vi "SaveImage.vi"(8 "error in (no error)":errorcluster caption="错误输入（无错误）", 9 "pSaveParam In":T1, 10 "pDstBuffer In":u8[](array[numeric]), 11 "pSrcData":u8[](array[numeric])) -> (0 "error out":errorcluster caption="错误输出", 1 "pSaveParam Out":T1, 2 "pDstBuffer Out":u8[](array[numeric]), 3 "function return":i32)   [LabVIEW 2015, in "MvCameraControl.lvlib"]
doc: "MV_LV_API int __stdcall SaveImage(MV_SAVE_IMAGE_PARAM* pSaveParam);"
uses:
  MvCameraControl.lvlib
  MvCameraPatch.dll
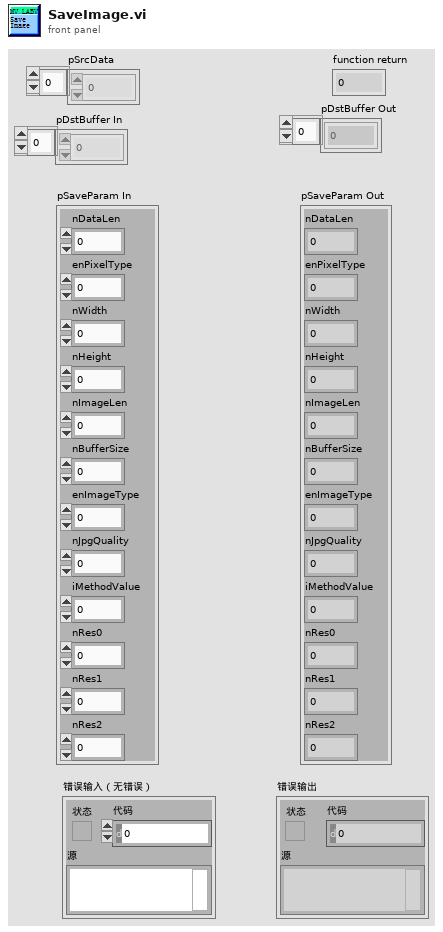
[diagram p1: front panel]
types:
  T1 = cluster{"nDataLen":u32, "enPixelType":i32, "nWidth":u16, "nHeight":u16, "nImageLen":u32, "nBufferSize":u32, "enImageType":u32, "nJpgQuality":u32, "iMethodValue":u32, "nRes0":u32, "nRes1":u32, "nRes2":u32}
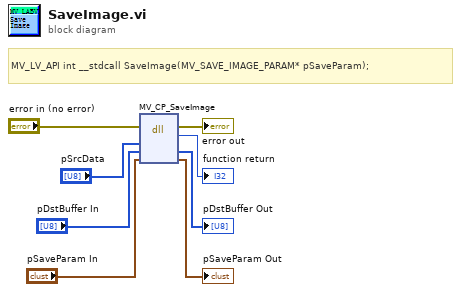
[diagram p0: block diagram]
diagram:
  # "MV_LV_API int __stdcall SaveImage(MV_SAVE_IMAGE_PARAM* pSaveParam);"
  n1 = dll-call lib="MvCameraPatch.dll" fn="MV_CP_SaveImage"(error in="error in (no error)", "pSrcData"="pSrcData", "pDstBuffer"="pDstBuffer In", "pSaveParam Out"="pSaveParam In") -> (error out=→"error out":errorcluster, "返回类型"=→"function return":i32, "pDstBuffer"=→"pDstBuffer Out":u8[], "pSaveParam Out"=→"pSaveParam Out":T1)  [unwired: 3 in, 1 out]
